vi "Set exposure mode.vi"(8 "error in (no error)":errorcluster, 10 "exposure mode":T1) -> (0 "error out":errorcluster, 2 "return value":i32)   [LabVIEW 2015]
doc: "Sets the exposure mode of the wavelength meter to either manual or automatic."
uses:
  HighFinesse WS5/Variable Typedefs.llb/Exposure Mode.ctl
  HighFinesse WS5/wlmData.dll
  HighFinesse WS5/HighFinesse WS5.lvlib
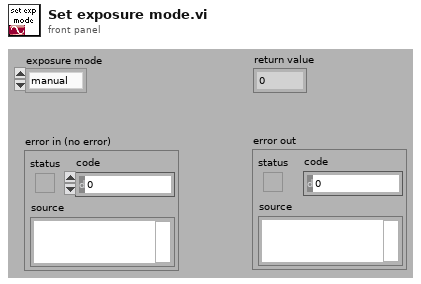
[diagram p1: front panel]
types:
  T1 = typedef "HighFinesse WS5.lvlib/Exposure Mode.ctl" = enum16{"manual", "automatic"}
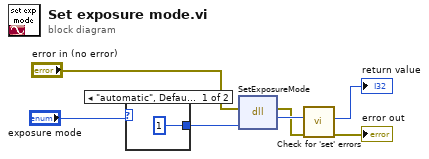
[diagram p0: block diagram]
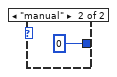
[diagram p2: hidden frame]
diagram:
  n1 = case shown="\"automatic\", Default" "exposure mode" {
    tunnel: [u8 1 u8 0] -> w2
    frame "automatic", Default {
    }
    frame "manual" {
    }
  }
  n2 = dll-call lib="C:/LabVIEW-programs-dev/Instruments/Wavelength meter/HighFinesse WS5/wlmData.dll" fn="SetExposureMode"(error in="error in (no error)", "EM"=w2) -> (error out=w4:errorcluster, "return value"=w6:i32)  [unwired: 3 in, 1 out]
  n3 = call "Check for 'set' errors.vi"("error in (no error)"=w4, "return value"=w6) -> ("error out"=→"error out":errorcluster, "return value out"=→"return value":i32)  [unwired: 8 out]
